vi "dragAndDrop.vi"() -> ()   [LabVIEW 2024]
uses:
  <vilib>/Utility/miscctls.llb/LVPoint32TypeDef.ctl
panel:
  out "led":bool
  in  "interruptor":bool
  in  "finalizar":bool
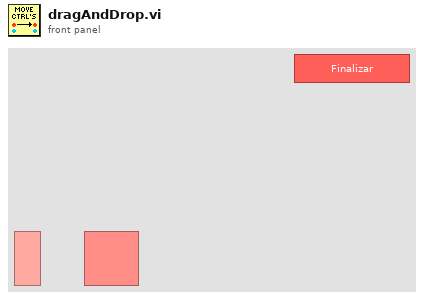
[diagram p1: front panel]
types:
  T1 = typedef "LVPoint32TypeDef.ctl" = cluster{"Horizontal":i32, "Vertical":i32}
  T2 = typedef "LVPositionTypeDef.ctl" = cluster{"Left":i32, "Top":i32}
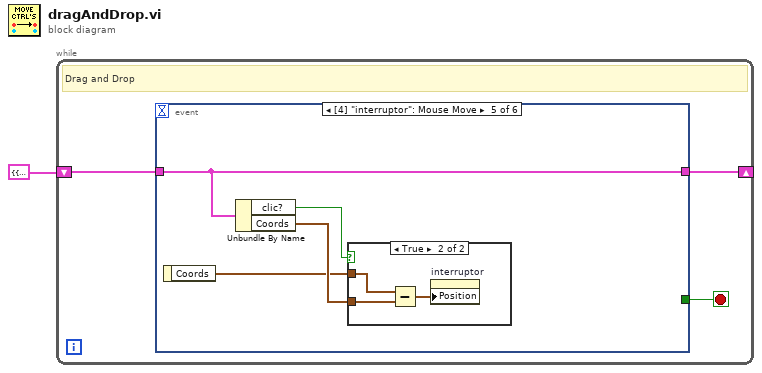
[diagram p0: block diagram]
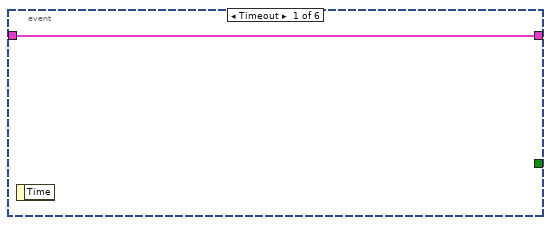
[diagram p2: hidden frame]
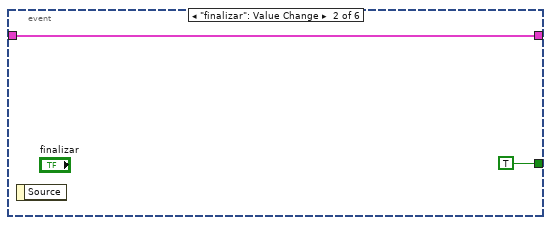
[diagram p3: hidden frame]
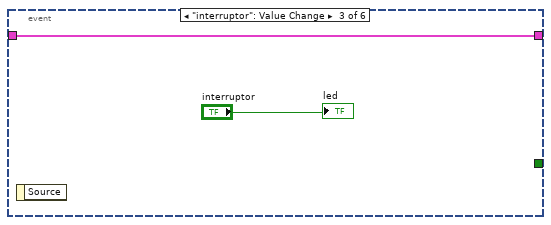
[diagram p4: hidden frame]
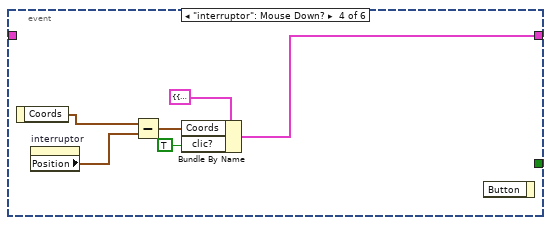
[diagram p5: hidden frame]
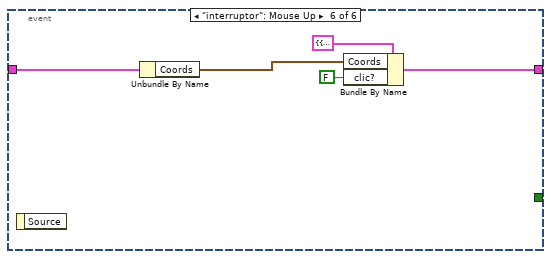
[diagram p7: hidden frame]
diagram:
  n1 = while {
    shift-right: [w4] -> _
    shift-left: cluster{"Coords":T1, "clic?":bool} {"Coords"={"Horizontal"=0, "Vertical"=0}, "clic?"=FALSE} -> [w3]
    stop <- w2 stop-if-true
    # "Drag and Drop"
    n2 = event shown="[4] \"interruptor\": Mouse Move" {
      selector: _ -> [_ _ _ _ _ _]
      dyn-events: _ -> [_ _ _ _ _ _]
      timeout: _ -> [_ _ _ _ _ _]
      tunnel: [w5 w6 w9 w10 w16 w23] -> w4
      tunnel: w3 -> [w5 w6 w9 _ w16 w26]
      tunnel: [_ TRUE _ _ _ _] -> w2
      event Timeout {
        n3 = event-data() -> ()  [unwired: 1 in, 1 out]
      }
      event "finalizar": Value Change {
        n4 = event-data() -> ()  [unwired: 1 in, 1 out]
      }
      event "interruptor": Value Change {
        n5 = event-data() -> ()  [unwired: 1 in, 1 out]
        "led" <- "interruptor"
      }
      event "interruptor": Mouse Down? {
        n6 = event-data() -> ("Coords"=w15:T1)  [unwired: 1 in]
        n7 = property on="interruptor" class="Bool (strict)"() -> ("Position"=w14:T2)  [unwired: 2 in, 2 out]
        n8 = Subtract(x=w15, y=w14) -> (x-y=w12:T1)
        n9 = Bundle By Name(cluster=cluster{"Coords":T1, "clic?":bool} {"Coords"={"Horizontal"=0, "Vertical"=0}, "clic?"=FALSE}, "Coords"=w12, "clic?"=TRUE) -> (w10:cluster{"Coords":T1, "clic?":bool})
        n10 = event-data() -> ()  [unwired: 2 in, 1 out]
      }
      event "interruptor": Mouse Move {
        n11 = event-data() -> ("Coords"=w17:T1)  [unwired: 1 in]
        n12 = Unbundle By Name(w16) -> ("clic?"=w18:bool, "Coords"=w19:T1)
        n13 = case shown="True" w18 {
          tunnel: w17 -> [_ w22]
          tunnel: w19 -> [_ w21]
          frame False {
          }
          frame True {
            n14 = Subtract(x=w22, y=w21) -> (x-y=w20:T1)
            n15 = property on="interruptor" class="Bool (strict)"("Position"=w20) -> ()  [unwired: 2 in, 2 out]
          }
        }
      }
      event "interruptor": Mouse Up {
        n16 = event-data() -> ()  [unwired: 1 in, 1 out]
        n17 = Unbundle By Name(w26) -> ("Coords"=w25:T1)
        n18 = Bundle By Name(cluster=cluster{"Coords":T1, "clic?":bool} {"Coords"={"Horizontal"=0, "Vertical"=0}, "clic?"=FALSE}, "Coords"=w25, "clic?"=FALSE) -> (w23:cluster{"Coords":T1, "clic?":bool})
      }
    }
  }
